vi "Calculate Component ID.vi"(11 "Input":string) -> (3 "Component ID":string)   [LabVIEW 2013, in "Attribute.Identity.lvclass"]
uses:
  Attribute.Identity.lvclass
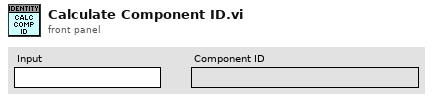
[diagram p1: front panel]
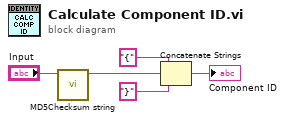
[diagram p0: block diagram]
diagram:
  n1 = call <vilib>:"MD5Checksum string.vi"("Message String"="Input") -> ("MD5 message-digest"=w2:string)  [unwired: 10 in]
  n2 = Concatenate Strings("{", w2, "}") -> (→"Component ID":string)
